vi "Write.vi"(8 "error in (no error)":errorcluster, 10 "Input":variant, 11 "Simulated HW in":refnum<class "Simulated HW.lvclass">) -> (0 "error out":errorcluster, 3 "Simulated HW out":refnum<class "Simulated HW.lvclass">)   [LabVIEW 2017, in "Simulated HW.lvclass"]
uses:
  Simulated HW.lvclass
  C:/Microcellular Plastics Lab/Hardware Settings/Hardware Types/Generic/Generic Hardware.lvclass
  Generic/Generic Hardware.lvclass/Generic Hardware.ctl
  Type Defs/Hardware Types.ctl
  Generic/Accessors/Read Description.vi
  Simulated HW Control Panel.vi
  Hardware Settings.lvclass
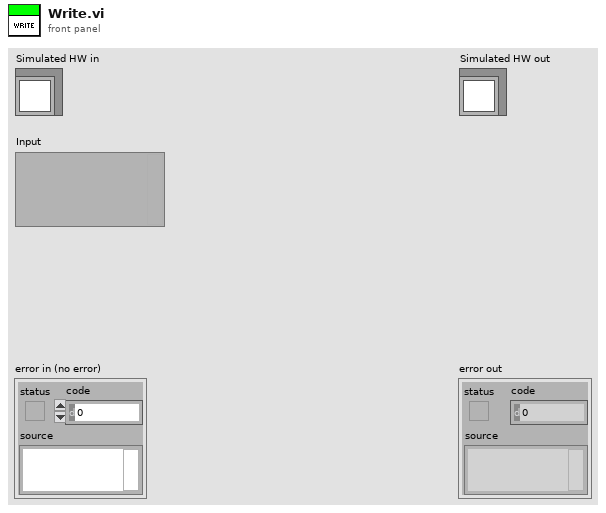
[diagram p1: front panel]
types:
  T1 = typedef "Hardware Settings.lvclass/Hardware Types.ctl" = string
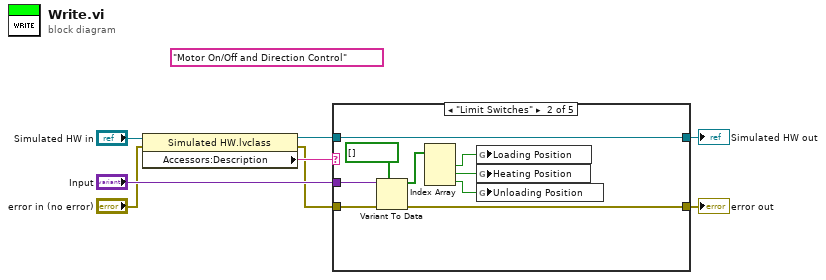
[diagram p0: block diagram]
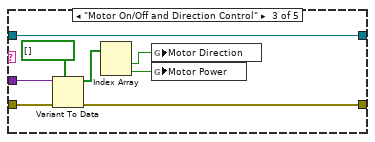
[diagram p3: hidden frame]
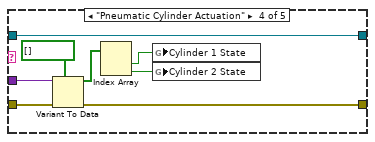
[diagram p4: hidden frame]
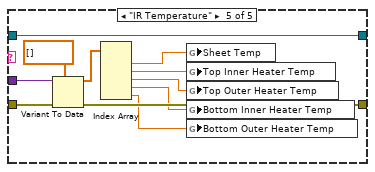
[diagram p5: hidden frame]
diagram:
  (unwired) T1 "Motor On/Off and Direction Control" ("Description")
  n1 = property class="Simulated HW.lvclass"(reference="Simulated HW in", error in="error in (no error)") -> (reference out=w1:refnum<class "Simulated HW.lvclass">, error out=w3:errorcluster, "Accessors:Description"=w6:T1)
  n2 = case shown="\"Limit Switches\"" w6 {
    tunnel: w3 -> [w10 w12 w21 w29 w40]
    tunnel: "Input" -> [_ w16 w25 w33 w44]
    tunnel: [w10 w11 w20 w28 w39] -> w5
    tunnel: [w9 w13 w22 w30 w41] -> w2
    tunnel: w1 -> [w9 w13 w22 w30 w41]
    frame "", Default {
    }
    frame "Limit Switches" {
      n3 = Variant To Data(error in=w12, type=bool[] [], Variant=w16) -> (data=w15:bool[], error out=w11:errorcluster)
      n4 = Index Array(array=w15) -> (element #1=w19:bool, element #2=w18:bool, element #3=w17:bool)  [unwired: 3 in]
      n5 = global write "Simulated HW Control Panel.vi" "Loading Position"(w19) -> ()
      n6 = global write "Simulated HW Control Panel.vi" "Heating Position"(w18) -> ()
      n7 = global write "Simulated HW Control Panel.vi" "Unloading Position"(w17) -> ()
    }
    frame "Motor On/Off and Direction Control" {
      n8 = Variant To Data(error in=w21, type=bool[] [], Variant=w25) -> (data=w24:bool[], error out=w20:errorcluster)
      n9 = Index Array(array=w24) -> (element #1=w27:bool, element #2=w26:bool)  [unwired: 2 in]
      n10 = global write "Simulated HW Control Panel.vi" "Motor Direction"(w27) -> ()
      n11 = global write "Simulated HW Control Panel.vi" "Motor Power"(w26) -> ()
    }
    frame "Pneumatic Cylinder Actuation" {
      n12 = Variant To Data(error in=w29, type=bool[] [], Variant=w33) -> (data=w32:bool[], error out=w28:errorcluster)
      n13 = Index Array(array=w32) -> (element #1=w35:bool, element #2=w34:bool)  [unwired: 2 in]
      n14 = global write "Simulated HW Control Panel.vi" "Cylinder 1 State"(w35) -> ()
      n15 = global write "Simulated HW Control Panel.vi" "Cylinder 2 State"(w34) -> ()
    }
    frame "IR Temperature" {
      n16 = Variant To Data(error in=w40, type=dbl[] [], Variant=w44) -> (data=w43:dbl[], error out=w39:errorcluster)
      n17 = Index Array(array=w43) -> (element #1=w46:dbl, element #2=w45:dbl, element #3=w38:dbl, element #4=w37:dbl, element #5=w36:dbl)  [unwired: 5 in]
      n18 = global write "Simulated HW Control Panel.vi" "Sheet Temp"(w46) -> ()
      n19 = global write "Simulated HW Control Panel.vi" "Top Inner Heater Temp"(w45) -> ()
      n20 = global write "Simulated HW Control Panel.vi" "Top Outer Heater Temp"(w38) -> ()
      n21 = global write "Simulated HW Control Panel.vi" "Bottom Inner Heater Temp"(w37) -> ()
      n22 = global write "Simulated HW Control Panel.vi" "Bottom Outer Heater Temp"(w36) -> ()
    }
  }
  "error out" <- w5
  "Simulated HW out" <- w2
